vi "GetBlobROI.vi"(2 "Dimension":i32=20, 3 "Centroid":cluster{"X":dbl, "Y":dbl}) -> (0 "Top Left":cluster{dbl, dbl}, 1 "ROI":T1)   [LabVIEW 2024]
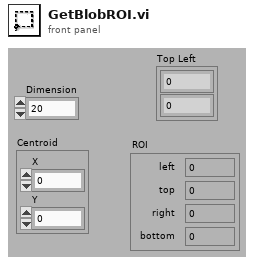
[diagram p1: front panel]
types:
  T1 = cluster{"left":i16, "top":i16, "right":i16, "bottom":i16}
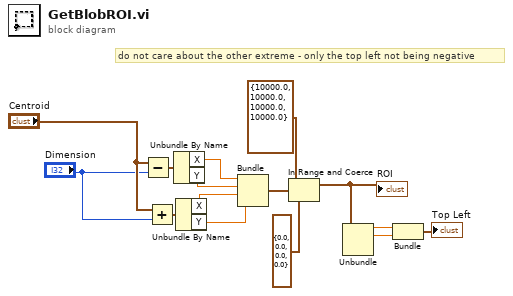
[diagram p0: block diagram]
diagram:
  # "do not care about the other extreme - only the top left not being negative"
  n1 = Subtract(x="Centroid", y="Dimension") -> (x-y=w14:cluster{"X":dbl, "Y":dbl})
  n2 = Add(x="Centroid", y="Dimension") -> (x+y=w11:cluster{"X":dbl, "Y":dbl})
  n3 = Unbundle By Name(w14) -> ("X"=w13:dbl, "Y"=w12:dbl)
  n4 = Unbundle By Name(w11) -> ("X"=w10:dbl, "Y"=w9:dbl)
  n5 = Bundle("X"=w13, "Y"=w12, "X"=w10, "Y"=w9) -> (w8:cluster{"X":dbl, "Y":dbl, "X":dbl, "Y":dbl})  [unwired: 1 in]
  n6 = In Range and Coerce(upper limit=cluster{"X":dbl, "Y":dbl, "X":dbl, "Y":dbl} {"X"=10000.0, "Y"=10000.0, "X"=10000.0, "Y"=10000.0}, x=w8, lower limit=cluster{"X":dbl, "Y":dbl, "X":dbl, "Y":dbl} {"X"=0.0, "Y"=0.0, "X"=0.0, "Y"=0.0}) -> (coerced(x)=w5:cluster{"X":dbl, "Y":dbl, "X":dbl, "Y":dbl})  [unwired: 1 out]
  "ROI" <- w5
  n7 = Unbundle(w5) -> ("X"=w4:dbl, "Y"=w3:dbl)  [unwired: 2 out]
  n8 = Bundle("X"=w4, "Y"=w3) -> (→"Top Left":cluster{"X":dbl, "Y":dbl})  [unwired: 1 in]
